vi "MTS_DrawCrossIMAQIamge.vi"(0 "Image":T1, 1 "Size":dbl=3.0, 2 "Color":u32, 5 "X":dbl, 7 "Y":dbl, 11 "error in (no error)":errorcluster) -> (4 "Image Out":T1, 15 "error out":errorcluster)   [LabVIEW 2011]
uses:
  <vilib>/vision/NI_Vision_Development_Module.lvlib
  <vilib>/vision/Image Controls.llb/IMAQ Image.ctl
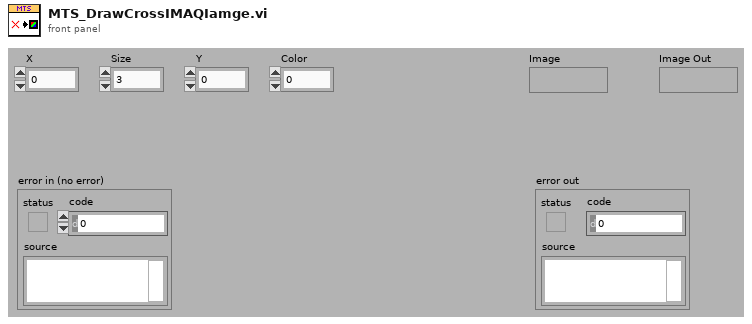
[diagram p1: front panel]
types:
  T1 = typedef "IMAQ Image.ctl" = refnum<image>
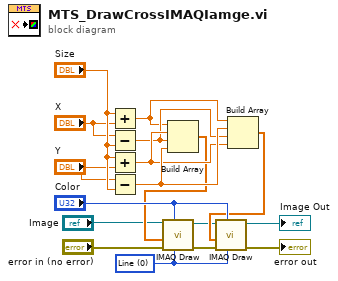
[diagram p0: block diagram]
diagram:
  w15 = u16 0 items=["Line", "Rectangle", "Oval"] ("Shape to draw")
  n1 = Add(x="Size", y="X") -> (x+y=w10:dbl)
  n2 = Subtract(x="X", y="Size") -> (x-y=w11:dbl)
  n3 = Add(x="Size", y="Y") -> (x+y=w12:dbl)
  n4 = Subtract(x="Y", y="Size") -> (x-y=w13:dbl)
  n5 = Build Array(w10, w12, w11, w13) -> (w9:dbl[])
  n6 = call "IMAQ Draw"("Shape to draw"=w15, "Pixel Color"="Color", "error in (no error)"="error in (no error)", "Coordinates"=w9, "Image Src"="Image") -> ("error out"=w2:errorcluster, "Image Dst Out"=w4:T1)  [unwired: 5 in]
  n7 = Build Array(w10, w13, w11, w12) -> (w14:dbl[])
  n8 = call "IMAQ Draw"("Shape to draw"=w15, "Pixel Color"="Color", "error in (no error)"=w2, "Coordinates"=w14, "Image Src"=w4) -> ("error out"=→"error out":errorcluster, "Image Dst Out"=→"Image Out":T1)  [unwired: 5 in]
